vi "update status.vi"(8 "error in (no error)":errorcluster, 10 "String In":string, 11 "LineCCD in":refnum<class "LineCCD.lvclass">) -> (0 "error out":errorcluster, 3 "LineCCD out":refnum<class "LineCCD.lvclass">)   [LabVIEW 2012, in "LineCCD.lvclass"]
uses:
  LineCCD.lvclass
  LineCCD.lvclass/LineCCD.ctl
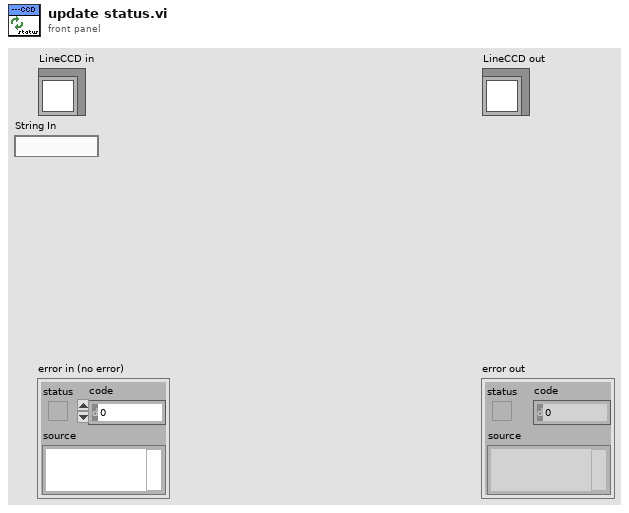
[diagram p1: front panel]
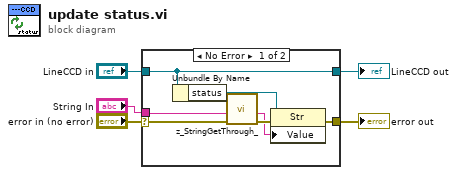
[diagram p0: block diagram]
diagram:
  n1 = case shown="No Error" "error in (no error)" {
    selector: "error in (no error)" -> [w12 w14]
    tunnel: [w8 w14] -> w4
    tunnel: [w11 w13] -> w2
    tunnel: "LineCCD in" -> [w11 w13]
    tunnel: "String In" -> [w6 _]
    frame No Error {
      n2 = Unbundle By Name(w11) -> ("status"=w10:refnum<vi>)
      n3 = call <instrlib>:"z_StringGetThrough_.vi"("Error In"=w12, "String In"=w6) -> ("Error Out"=w9:errorcluster, "String Out"=w7:string)  [unwired: 8 in]
      n4 = property class="Str"(reference=w10, error in=w9, "Value"=w7) -> (error out=w8:errorcluster)  [unwired: 1 out]
    }
    frame Error {
    }
  }
  "error out" <- w4
  "LineCCD out" <- w2
